vi "Fetch Waveform Measurement.vi"(7 "Destination Channel (1: Channel 2)":u16(ring)=1 items=["Channel 1", "Channel 2", "Channel 3", "Channel 4", "Math", "D0", "D1", "D2", "D3", "D4", "D5", "D6", "D7", "D8", "D9", "D10", "D11", "D12", "D13", "D14", "D15", "Reference 1", "Reference 2", "Reference 3", "Reference 4", "Amplitude", "Frequency", "Phase"], 8 "error in (no error)":errorcluster, 9 "Measurement Function (0: Period)":i32(ring) items=["Period", "Frequency", "Delay", "Rise Time", "Fall Time", "Positive Duty Cycle", "Negative Duty Cycle", "Positive Pulse Width", "Negative Pulse Width", "Burst Width", "Phase", "Positive Overshoot", "Negative Overshoot", "Vpp", "Amplitude", "Voltage High", "Voltage Low", "Voltage Max", "Voltage Min", "Voltage Mean", "Voltage Mean (cycle)", "Voltage RMS", "Voltage RMS (cycle)", "Area", "Cycle Area", "Positive Edge Count", "Negative Edge Count", "Positive Pulse Count", "Negative Pulse Count"], 10 "Channel (0: Channel 1)":u16(ring) items=["Channel 1", "Channel 2", "Channel 3", "Channel 4", "Math", "D0", "D1", "D2", "D3", "D4", "D5", "D6", "D7", "D8", "D9", "D10", "D11", "D12", "D13", "D14", "D15", "Reference 1", "Reference 2", "Reference 3", "Reference 4", "Amplitude", "Frequency", "Phase"], 11 "VISA resource name":refnum<visa-resource-name>) -> (0 "error out":errorcluster, 2 "Measurement Value":dbl, 3 "VISA resource name out":refnum<visa-resource-name>)   [LabVIEW 2010, in "Tektronix DPO MSO 2000 4000 Series.lvlib"]
doc: "Initiates an acquisition on the channel that you specify in the <B>Channel</B> control. After the acquisition completes, the Fetch Waveform Measurement VI performs waveform measurement on the channel you specify and returns a measurement value. You can specify a measurement type, such as rise time, frequency, and voltage peak-to-peak, with this VI. Use the Fetch Waveform Measurement VI separately for any other waveform measurement on a channel without initiating another acquisition."
uses:
  <instrlib>/Tektronix DPO MSO 2000 4000 Series/Tektronix DPO MSO 2000 4000 Series.lvlib
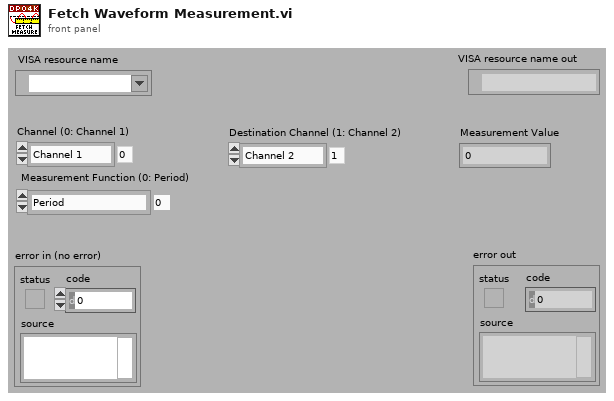
[diagram p1: front panel]
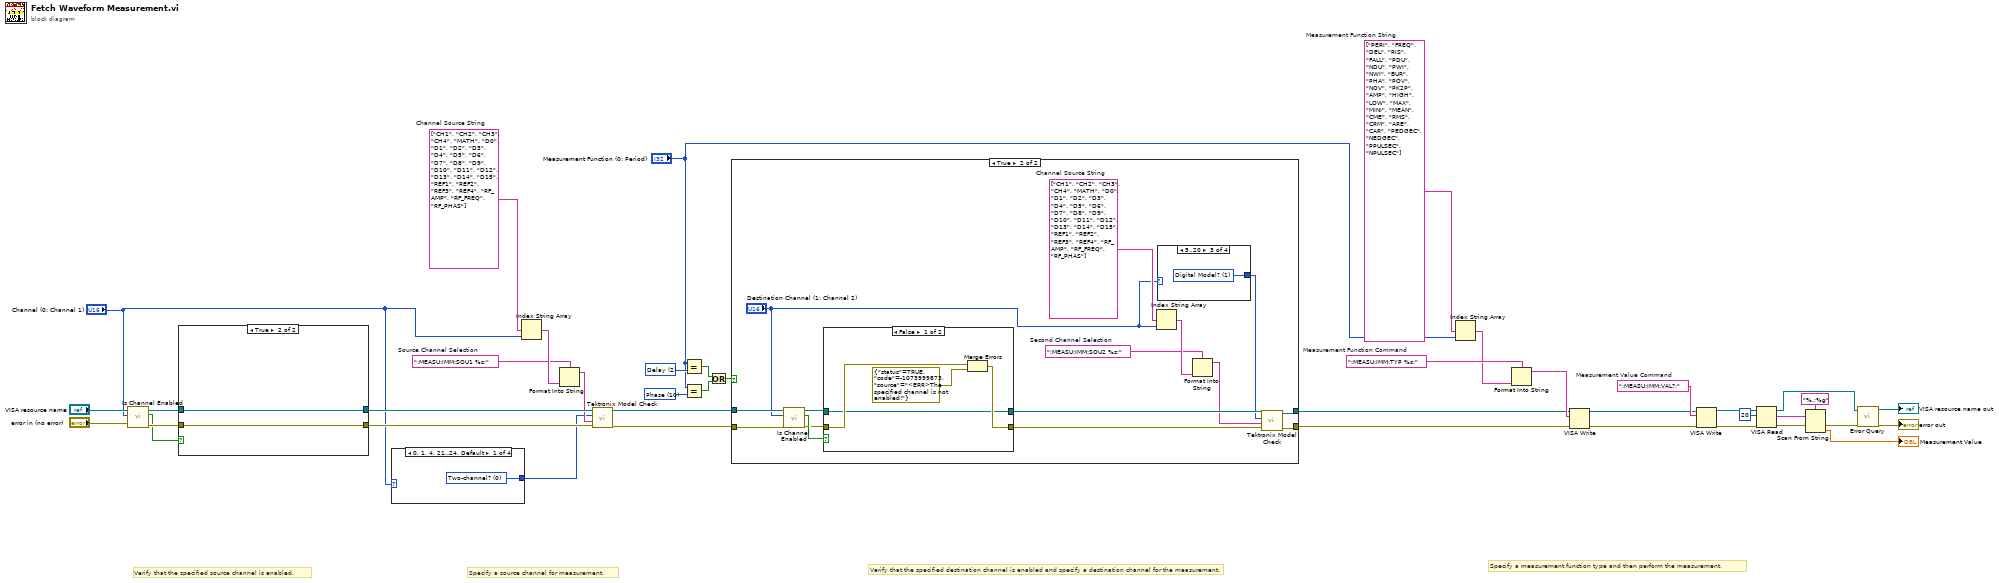
[diagram p0: block diagram]
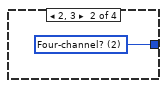
[diagram p2: hidden frame]
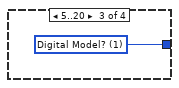
[diagram p3: hidden frame]
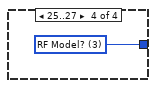
[diagram p4: hidden frame]
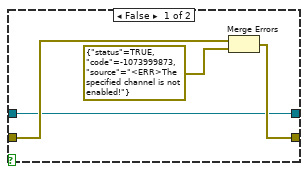
[diagram p5: hidden frame]
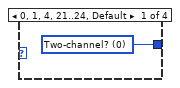
[diagram p7: hidden frame]
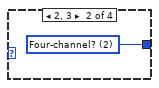
[diagram p8: hidden frame]
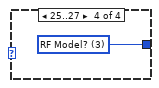
[diagram p9: hidden frame]
diagram:
  w12 = ":MEASU:IMM:SOU1 %s;"  # Source Channel Selection
  w11 = string[] ["CH1", "CH2", "CH3", "CH4", "MATH", "D0", "D1", "D2", "D3", "D4", "D5", "D6", "D7", "D8", "D9", "D10", "D11", "D12", "D13", "D14", "D15", "REF1", "REF2", "REF3", "REF4", "RF_AMP", "RF_FREQ", "RF_PHAS"]  # Channel Source String
  w29 = ":MEASU:IMM:VAL?;"  # Measurement Value Command
  w37 = u16 10 items=["Period", "Frequency", "Delay", "Rise Time", "Fall Time", "Positive Duty Cycle", "Negative Duty Cycle", "Positive Pulse Width", "Negative Pulse Width", "Burst Width", "Phase", "Positive Overshoot", "Negative Overshoot", "Pk-Pk", "Amplitude", "High", "Low", "Max", "Min", "Mean", "Cycle Mean", "RMS", "Cycle RMS", "Area", ""]
  w38 = u16 2 items=["Period", "Frequency", "Delay", "Rise Time", "Fall Time", "Positive Duty Cycle", "Negative Duty Cycle", "Positive Pulse Width", "Negative Pulse Width", "Burst Width", "Phase", "Positive Overshoot", "Negative Overshoot", "Pk-Pk", "Amplitude", "High", "Low", "Max", "Min", "Mean", "Cycle Mean", "RMS", "Cycle RMS", "Area", ""]
  w40 = ":MEASU:IMM:TYP %s;"  # Measurement Function Command
  w41 = string[] ["PERI", "FREQ", "DEL", "RIS", "FALL", "PDU", "NDU", "PWI", "NWI", "BUR", "PHA", "POV", "NOV", "PK2P", "AMP", "HIGH", "LOW", "MAX", "MINI", "MEAN", "CME", "RMS", "CRM", "ARE", "CAR", "PEDGEC", "NEDGEC", "PPULSEC", "NPULSEC"]  # Measurement Function String
  # "Specify a measurement function type and then perform the measurement."
  # "Verify that the specified destination channel is enabled and specify a destination channel for the measurement."
  # "Specify a source channel for measurement."
  # "Verify that the specified source channel is enabled."
  n1 = call <instrlib>:"Is Channel Enabled.vi"("error in (no error)"="error in (no error)", "Channel (0: Channel 1)"="Channel (0: Channel 1)", "VISA resource name"="VISA resource name") -> ("error out"=w15:errorcluster, "Enabled"=w14:bool, "VISA resource name out"=w16:refnum<visa-resource-name>)  [unwired: 6 in]
  n2 = case shown="True" w14 {
    tunnel: w16 -> [w42 w47]
    tunnel: w15 -> [w44 w46]
    tunnel: [w42 w47] -> w7
    tunnel: [w43 w46] -> w6
    frame False {
      n3 = Merge Errors(w44, errorcluster {"status"=TRUE, "code"=-1073999873, "source"="<ERR>The specified channel is not enabled!"} ("error out")) -> (w43:errorcluster)
    }
    frame True {
    }
  }
  n4 = case shown="0, 1, 4, 21..24, Default" "Channel (0: Channel 1)" {
    tunnel: [w48 w49 w50 w51] -> w1
    frame 0, 1, 4, 21..24, Default {
      w48 = u16 0 items=["Two-channel?", "Digital Model?", "Four-channel?", "RF Model?"] ("Oscilloscope Model Tests (3: RF Model?)")
    }
    frame 2, 3 {
      w49 = u16 2 items=["Two-channel?", "Digital Model?", "Four-channel?", "RF Model?"] ("Oscilloscope Model Tests (3: RF Model?)")
    }
    frame 5..20 {
      w50 = u16 1 items=["Two-channel?", "Digital Model?", "Four-channel?", "RF Model?"] ("Oscilloscope Model Tests (3: RF Model?)")
    }
    frame 25..27 {
      w51 = u16 3 items=["Two-channel?", "Digital Model?", "Four-channel?", "RF Model?"] ("Oscilloscope Model Tests (3: RF Model?)")
    }
  }
  n5 = Index String Array(1:"Channel (0: Channel 1)", 2:w11) -> (0:w13:string)  [unwired: 1 in]
  n6 = Format Into String(format string=w12, w13) -> (resulting string=w5:string)  [unwired: 2 in, 1 out]
  n7 = call <instrlib>:"Tektronix Model Check.vi"("error in (no error)"=w6, "Command String"=w5, "Oscilloscope Model Tests (3: RF Model?)"=w1, "VISA resource name"=w7) -> ("error out"=w3:errorcluster, "VISA resource name out"=w4:refnum<visa-resource-name>)  [unwired: 6 in]
  n8 = Equal?(x="Measurement Function (0: Period)", y=w38) -> (x = y?=w36:bool)
  n9 = Equal?(x="Measurement Function (0: Period)", y=w37) -> (x = y?=w35:bool)
  n10 = Or(x=w36, y=w35) -> (x .or. y?=w34:bool)
  n11 = case shown="True" w34 {
    tunnel: w4 -> [w53 w66]
    tunnel: w3 -> [w52 w65]
    tunnel: [w53 w57] -> w31
    tunnel: [w52 w56] -> w30
    frame False {
    }
    frame True {
      w61 = string[] ["CH1", "CH2", "CH3", "CH4", "MATH", "D0", "D1", "D2", "D3", "D4", "D5", "D6", "D7", "D8", "D9", "D10", "D11", "D12", "D13", "D14", "D15", "REF1", "REF2", "REF3", "REF4", "RF_AMP", "RF_FREQ", "RF_PHAS"]  # Channel Source String
      w67 = ":MEASU:IMM:SOU2 %s;"  # Second Channel Selection
      n12 = call <instrlib>:"Is Channel Enabled.vi"("error in (no error)"=w65, "Channel (0: Channel 1)"="Destination Channel (1: Channel 2)", "VISA resource name"=w66) -> ("error out"=w62:errorcluster, "Enabled"=w64:bool, "VISA resource name out"=w63:refnum<visa-resource-name>)  [unwired: 6 in]
      n13 = case shown="False" w64 {
        tunnel: w63 -> [w73 w78]
        tunnel: w62 -> [w75 w77]
        tunnel: [w73 w78] -> w60
        tunnel: [w74 w77] -> w59
        frame False {
          n14 = Merge Errors(w75, errorcluster {"status"=TRUE, "code"=-1073999873, "source"="<ERR>The specified channel is not enabled!"} ("error out")) -> (w74:errorcluster)
        }
        frame True {
        }
      }
      n15 = Index String Array(1:"Destination Channel (1: Channel 2)", 2:w61) -> (0:w68:string)  [unwired: 1 in]
      n16 = case shown="5..20" "Destination Channel (1: Channel 2)" {
        tunnel: [w69 w70 w71 w72] -> w54
        frame 0, 1, 4, 21..24, Default {
          w69 = u16 0 items=["Two-channel?", "Digital Model?", "Four-channel?", "RF Model?"] ("Oscilloscope Model Tests (3: RF Model?)")
        }
        frame 2, 3 {
          w70 = u16 2 items=["Two-channel?", "Digital Model?", "Four-channel?", "RF Model?"] ("Oscilloscope Model Tests (3: RF Model?)")
        }
        frame 5..20 {
          w71 = u16 1 items=["Two-channel?", "Digital Model?", "Four-channel?", "RF Model?"] ("Oscilloscope Model Tests (3: RF Model?)")
        }
        frame 25..27 {
          w72 = u16 3 items=["Two-channel?", "Digital Model?", "Four-channel?", "RF Model?"] ("Oscilloscope Model Tests (3: RF Model?)")
        }
      }
      n17 = Format Into String(format string=w67, w68) -> (resulting string=w58:string)  [unwired: 2 in, 1 out]
      n18 = call <instrlib>:"Tektronix Model Check.vi"("error in (no error)"=w59, "Command String"=w58, "Oscilloscope Model Tests (3: RF Model?)"=w54, "VISA resource name"=w60) -> ("error out"=w56:errorcluster, "VISA resource name out"=w57:refnum<visa-resource-name>)  [unwired: 6 in]
    }
  }
  n19 = Index String Array(1:"Measurement Function (0: Period)", 2:w41) -> (0:w39:string)  [unwired: 1 in]
  n20 = Format Into String(format string=w40, w39) -> (resulting string=w33:string)  [unwired: 2 in, 1 out]
  n21 = VISA Write(VISA resource name=w31, write buffer=w33, error in (no error)=w30) -> (VISA resource name out=w22:refnum<visa-resource-name>, error out=w21:errorcluster)  [unwired: 1 out]
  n22 = VISA Write(VISA resource name=w22, write buffer=w29, error in (no error)=w21) -> (VISA resource name out=w28:refnum<visa-resource-name>, error out=w27:errorcluster)  [unwired: 1 out]
  n23 = VISA Read(VISA resource name=w28, byte count=u32 20, error in (no error)=w27) -> (VISA resource name out=w8:refnum<visa-resource-name>, read buffer=w25:string, error out=w10:errorcluster)  [unwired: 1 out]
  n24 = Scan From String(format string="%.;%g", input string=w25, error in=w10) -> (error out=w9:errorcluster, output 1=→"Measurement Value":dbl)  [unwired: 2 in, 2 out]
  n25 = call <instrlib>:"Error Query.vi"("error in (no error)"=w9, "VISA resource name"=w8) -> ("error out"=→"error out":errorcluster, "VISA resource name out"=→"VISA resource name out":refnum<visa-resource-name>)  [unwired: 6 in, 2 out]
